vi "AddDevice.vi"(0 "Device List in":refnum<class "Device.lvclass">[](array[class]), 1 "Table Ref In":refnum<vi>, 2 "Table History ref":refnum<vi>, 3 "Layout Ref":refnum<vi>, 5 "DevNums In":i32[](array[numeric]), 9 "Col array in":refnum<class "Column.lvclass">[](array[class]), 11 "error in (no error)":errorcluster, 12 "Add Device":refnum<vi>) -> (4 "Device List out":refnum<class "Device.lvclass">[](array[class]), 6 "DevNums Out":i32[](array[numeric]), 10 "Col array out":refnum<class "Column.lvclass">[](array[class]), 14 "Changes Made?":bool, 15 "error out":errorcluster)   [LabVIEW 2013]
doc: "Add user selected device (based on typedef AddDeviceRing.ctl!).\nUpdates Device object array, table Col array, DevNums array AND pushes appearance update to table.\n\nClearly, this VI requires read/write access to column array."
uses:
  Device/Device.lvclass
  ColumnVIs/Column/Column.lvclass
  TypeDefs/AddDeviceRing.ctl
  TypeDefs/TableHistory.ctl
  TypeDefs/TableArray.ctl
  DDS/DDS.lvclass
  Novatech/Novatech.lvclass
  NI Card/NI Card.lvclass
  Slave_Pulseblaster/Slave_Pulseblaster.lvclass
  PTS-via-PB/PTS-via-PB.lvclass
  Master Device/Master Device.lvclass
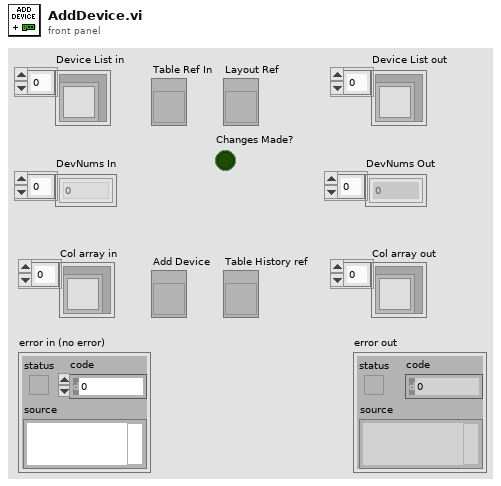
[diagram p1: front panel]
types:
  T1 = typedef "AddDeviceRing.ctl" = u16
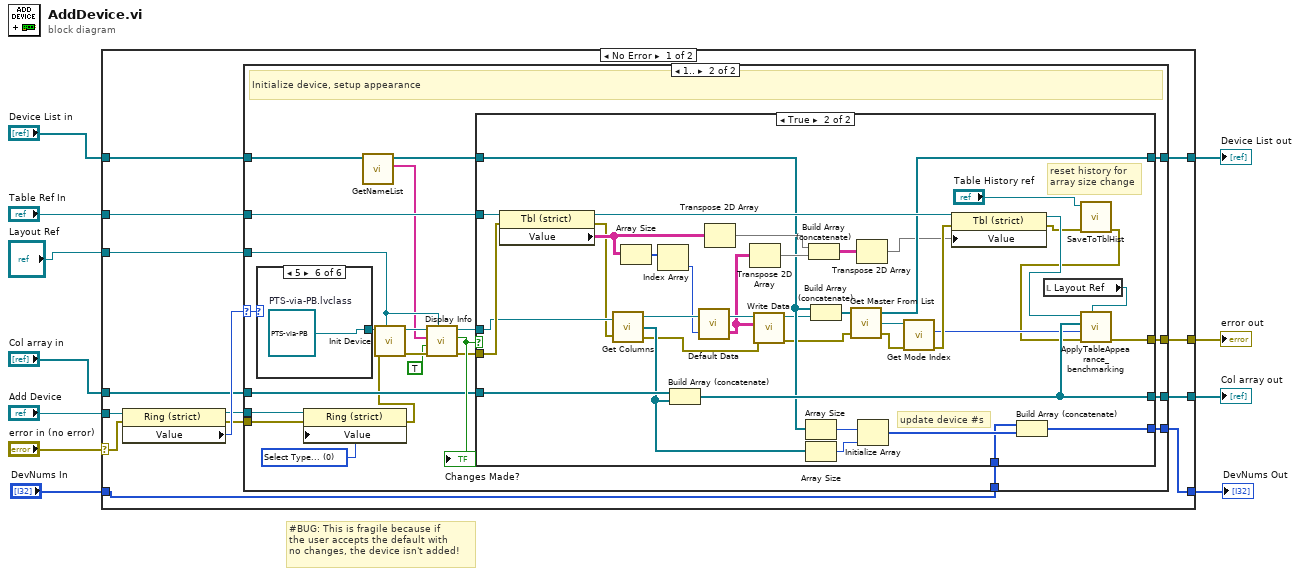
[diagram p0: block diagram]
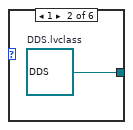
[diagram p5: hidden frame]
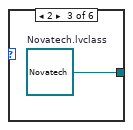
[diagram p6: hidden frame]
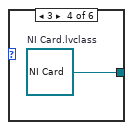
[diagram p7: hidden frame]
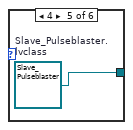
[diagram p8: hidden frame]
diagram:
  # "#BUG: This is fragile because if \nthe user accepts the default with\nno changes, the device isn't added!"
  n1 = case shown="No Error" "error in (no error)" {
    selector: "error in (no error)" -> [w24 w102]
    tunnel: "Add Device" -> [w25 _]
    tunnel: "Table Ref In" -> [w20 _]
    tunnel: "Device List in" -> [w19 w104]
    tunnel: [w18 w104] -> w7
    tunnel: "Col array in" -> [w17 w103]
    tunnel: [w16 w103] -> w5
    tunnel: [w15 w102] -> w4
    tunnel: "DevNums In" -> [w14 w101]
    tunnel: [w13 w101] -> w2
    tunnel: "Layout Ref" -> [w12 _]
    frame No Error {
      n2 = property class="Ring (strict)"(reference=w25, error in=w24) -> (reference out=w21:refnum<vi>, error out=w22:errorcluster, "Value"=w23:u16)
      n3 = case shown="1.." w23 {
        selector: w23 -> [_ w49]
        tunnel: w22 -> [w27 w51]
        tunnel: w21 -> [_ w52]
        tunnel: w20 -> [_ w46]
        tunnel: w19 -> [w28 w33]
        tunnel: [w28 w44] -> w18
        tunnel: w17 -> [w29 w43]
        tunnel: [w29 w42] -> w16
        tunnel: [w27 w41] -> w15
        tunnel: w14 -> [w26 w40]
        tunnel: [w26 w39] -> w13
        tunnel: w12 -> [_ w36]
        frame 0, Default {
          # "0 is \"select type...\""
        }
        frame 1.. {
          w50 = T1 0 items=["Select Type...", "DDS", "Novatech", "NI Card"] ("Add Device 2")
          # "Initialize device, setup appearance"
          n4 = case shown="5" w49 {
            tunnel: [_ w96 w97 w98 w99 w100] -> w37
            frame Default {
            }
            frame 1 {
              w96 = refnum<class "DDS.lvclass"> refnum  # DDS.lvclass
            }
            frame 2 {
              w97 = refnum<class "Novatech.lvclass"> refnum  # Novatech.lvclass
            }
            frame 3 {
              w98 = refnum<class "NI Card.lvclass"> refnum  # NI Card.lvclass
            }
            frame 4 {
              w99 = refnum<class "Slave_Pulseblaster.lvclass"> refnum  # Slave_Pulseblaster.lvclass
            }
            frame 5 {
              w100 = refnum<class "PTS-via-PB.lvclass"> refnum  # PTS-via-PB.lvclass
            }
          }
          n5 = property class="Ring (strict)"(reference=w52, error in=w51, "Value"=w50) -> (error out=w34:errorcluster)  [unwired: 1 out]
          n6 = call "GetNameList.vi"("Devices"=w33) -> ("Names in use"=w31:string[], "Devices out"=w32:refnum<class "Device.lvclass">[])  [unwired: 8 in, 1 out]
          n7 = call-dynamic "Init Device.vi"("Layout Ref"=w36, "error in (no error)"=w34, "Device in"=w37) -> ("error out"=w35:errorcluster, "Device out"=w38:refnum<class "Device.lvclass">)  [unwired: 7 in]
          n8 = call-dynamic "Display Info.vi"("Layout ref"=w36, "error in (no error)"=w35, "Modify (F) /Add [T]"=TRUE, "Names in use"=w31, "Device in"=w38) -> ("error out"=w47:errorcluster, "Changes Made?"=w48:bool, "Device out"=w45:refnum<class "Device.lvclass">)  [unwired: 3 in, 1 out]
          "Changes Made?" <- w48
          n9 = case shown="True" w48 {
            tunnel: w47 -> [w54 w95]
            tunnel: w46 -> [_ w94]
            tunnel: w45 -> [_ w83]
            tunnel: w32 -> [w56 w73]
            tunnel: [w56 w80] -> w44
            tunnel: w43 -> [w55 w79]
            tunnel: [w55 w76] -> w42
            tunnel: [w54 w74] -> w41
            tunnel: w40 -> [w53 w68]
            tunnel: [w53 w67] -> w39
            frame False {
              # "User cancelled: pass through un-appended devices + columns"
            }
            frame True {
              # "reset history for\narray size change"
              # "update device #s"
              n10 = property class="Tbl (strict)"(reference=w94, error in=w95) -> (reference out=w93:refnum<vi>, error out=w82:errorcluster, "Value"=w84:string[][])
              n11 = call-dynamic "Get Columns.vi"("Device in"=w83, "error in (no error)"=w82) -> ("Device out"=w89:refnum<class "Device.lvclass">, "Columns"=w71:refnum<class "Column.lvclass">[], "error out"=w62:errorcluster)
              n12 = Array Size(array=w84) -> (size(s)=w88:i32[])
              n13 = Index Array(array=w88) -> (element=w87:i32)  [unwired: 1 in]
              n14 = Build Array (concatenate)(w79, w71) -> (w76:refnum<class "Column.lvclass">[])
              n15 = call-dynamic "Default Data.vi"("Num Rows"=w87, "Device in"=w89) -> ("Default Data"=w60:string[][], "Device out"=w64:refnum<class "Device.lvclass">)
              n16 = Transpose 2D Array(2D array=w84) -> (transposed array=w92:string[][])
              n17 = Transpose 2D Array(2D array=w60) -> (transposed array=w91:string[][])
              n18 = call-dynamic "Write Data.vi"("error in (no error)"=w62, "Data"=w60, "Device in"=w64) -> ("error out"=w61:errorcluster, "Device Out"=w63:refnum<class "Device.lvclass">)  [unwired: 7 in]
              n19 = Array Size(array=w73) -> (size(s)=w72:i32)
              n20 = Array Size(array=w71) -> (size(s)=w70:i32)
              n21 = Build Array (concatenate)(w92, w91) -> (w90:string[][])
              n22 = Build Array (concatenate)(w73, w63) -> (w86:refnum<class "Device.lvclass">[])
              n23 = call "Get Master From List.vi"("error in"=w61, "Device List in"=w86) -> ("error out"=w81:errorcluster, "Master Device"=w85:refnum<class "Master Device.lvclass">, "Device List out"=w80:refnum<class "Device.lvclass">[])  [unwired: 1 in]
              n24 = Transpose 2D Array(2D array=w90) -> (transposed array=w77:string[][])
              n25 = Initialize Array(w72, w70) -> (w69:i32[])
              n26 = call-dynamic "Get Mode Index.vi"("error in (no error)"=w81, "Master Device in"=w85) -> ("error out"=w78:errorcluster, "Mode Col"=w75:i32)  [unwired: 7 in, 1 out]
              n27 = property class="Tbl (strict)"(reference=w93, error in=w78, "Value"=w77) -> (reference out=w66:refnum<vi>, error out=w59:errorcluster)
              n28 = Build Array (concatenate)(w68, w69) -> (w67:i32[])
              n29 = local read "Layout Ref"() -> (w65:refnum<vi>)
              n30 = call "SaveToTblHist.vi"("error in (no error)"=w59, "Table History ref"="Table History ref") -> ("error out"=w58:errorcluster)  [unwired: 9 in]
              n31 = call "ApplyTableAppearance_benchmarking.vi"("Layout Ring Ref"=w65, "error in (no error)"=w58, "Mode Index"=w75, "Col Array in"=w76, "Table Ref in"=w66) -> ("error out"=w74:errorcluster)  [unwired: 5 in, 1 out]
            }
          }
        }
      }
    }
    frame Error {
    }
  }
  "Col array out" <- w5
  "error out" <- w4
  "Device List out" <- w7
  "DevNums Out" <- w2
